vi "Get Measurement Matrices.vi"(10 "Sensors":T3[](array[typedef]), 11 "System States":T2[](array[typedef])) -> (2 "R (Measurement Uncertainty)":T1, 3 "H (Observation Matrix)":T1)   [LabVIEW 2020]
uses:
  Sensor.ctl
  Sensor Type.ctl
  Measurement.ctl
  State.ctl
  <vilib>/Analysis/Matrix/Datatypes/RealMatrix.ctl
  <vilib>/Analysis/Matrix/Numeric/Conversions/Array To Matrix - RA2.vi
  <vilib>/Analysis/7linalg.llb/Create Special Real Matrix.vi
  <vilib>/Analysis/NI_AALPro.lvlib
  <vilib>/Analysis/Matrix/NI_Matrix.lvlib
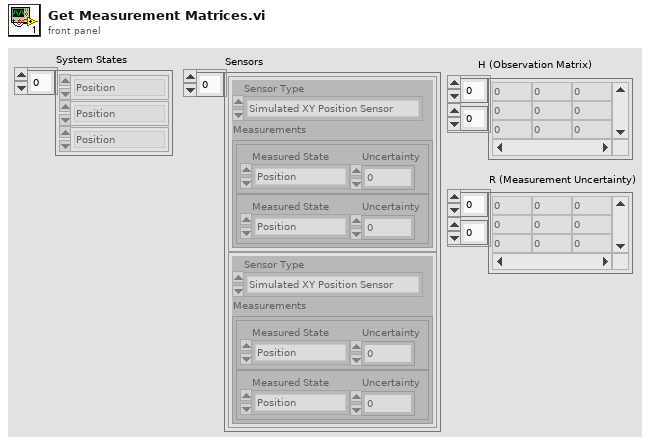
[diagram p1: front panel]
types:
  T1 = typedef "NI_Matrix.lvlib/RealMatrix.ctl" = dbl[][]
  T2 = typedef "State.ctl" = enum16{"Position", "Velocity"}
  T3 = typedef "Sensor.ctl" = cluster{"Sensor Type":T4, "Measurements":T5[]}
  T4 = typedef "Sensor Type.ctl" = enum16{"Simulated XY Position Sensor", "Simulated XY Velocity Sensor"}
  T5 = typedef "Measurement.ctl" = cluster{"Measured State":T2, "Uncertainty":dbl}
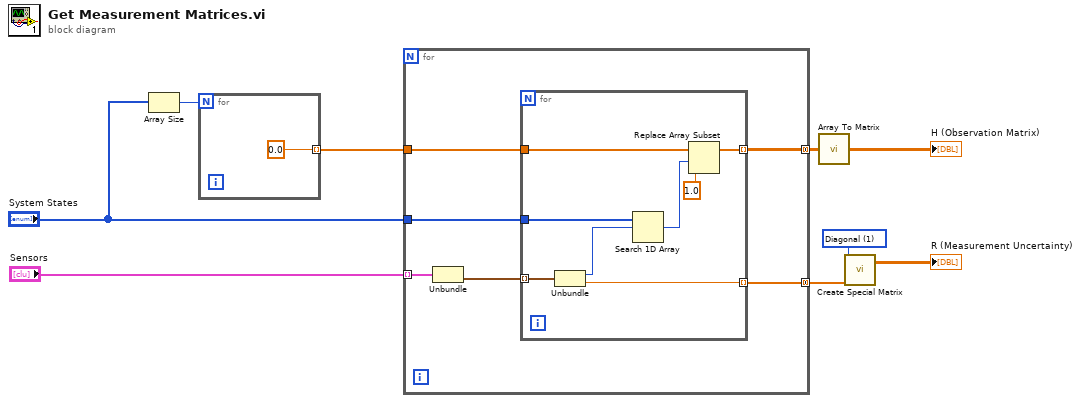
[diagram p0: block diagram]
diagram:
  w8 = 1 items=["Identity", "Diagonal", "Toeplitz", "Vandermonde", "Companion", "Hankel", "Hadamard", "Wilkinson", "Hilbert", "Inverse Hilbert", "Rosser", "Pascal"] ("matrix type")
  n1 = Array Size(array="System States") -> (size(s)=w5:i32)
  n2 = for {
    N: w5 -> [_]
    tunnel: [0.0] -> w3 mode=indexing
  }
  n3 = for {
    tunnel: "Sensors" -> [w16] mode=indexing
    tunnel: [w14] -> w7 mode=concatenating
    tunnel: "System States" -> [w13]
    tunnel: w3 -> [w12]
    tunnel: [w11] -> w2 mode=concatenating
    n4 = Unbundle(w16) -> ("Measurements"=w15:T5[])  [unwired: 1 out]
    n5 = for {
      tunnel: w15 -> [w24] mode=indexing
      tunnel: [w23] -> w14 mode=indexing
      tunnel: w13 -> [w21]
      tunnel: w12 -> [w20]
      tunnel: [w17] -> w11 mode=indexing
      n6 = Unbundle(w24) -> ("Measured State"=w22:T2, "Uncertainty"=w23:dbl)
      n7 = Search 1D Array(1D array=w21, element=w22) -> (index of element=w19:i32)  [unwired: 1 in]
      n8 = Replace Array Subset(array=w20, new element=1.0 ("new element/subarray"), index=w19) -> (w17:dbl[])
    }
  }
  n9 = call-poly <vilib>:"Array To Matrix.vi"("Real 2D Array"=w2) -> ("Real Matrix"=→"H (Observation Matrix)":T1)
  n10 = call-poly <vilib>:"Create Special Matrix.vi"("matrix type"=w8, "Input Vector1"=w7) -> ("Special Matrix"=→"R (Measurement Uncertainty)":T1)  [unwired: 3 in, 1 out]
